vi "Udp Tester ffwd P Deadband.vi"() -> ()   [LabVIEW 2014]
uses:
  <vilib>/Simulation/Scripting/Companion Diagram/SimConfigNode/SimParams.ctl
  <vilib>/Simulation/Scripting/Companion Diagram/SimConfigNode/_simSolvers.ctl
  <vilib>/Simulation/Implementation/Shared/SIMSCR Execution Mode.ctl
  <vilib>/Platform/TimedLoop/XDataNode/timing_clust.ctl
  <vilib>/Platform/TimedLoop/XDataNode/nitl_modes.ctl
  <vilib>/Platform/TimedLoop/XDataNode/wakeup.ctl
  <vilib>/Simulation/Param Hierarchy/Typedefs/SIMPH Param Control Actions.ctl
  <vilib>/Simulation/Scripting/Editor Utilities/SIM subVI tag data.ctl
  <vilib>/Simulation/Scripting/Editor Utilities/SIM subVI execution type.ctl
  <vilib>/Simulation/Implementation/Shared/NILVSim_ParamChanged.vi
  <vilib>/Simulation/Implementation/Shared/NILVSim_FinishedLate.vi
  <vilib>/Simulation/Implementation/Shared/NILVSIM_BeginStep.vi
  <vilib>/Simulation/Utility/Implementation/SIM Time.vi
  <vilib>/Simulation/SignalArithmetic/Implementation/NILVSim Gain.llb/SIM Gain (scalar).vi
  <vilib>/Simulation/DiscreteLinear/Implementation/NILVSim Discrete Integrator Forward.llb/SIM Discrete Integrator Forward Distributor (scalar).vi
  <vilib>/Simulation/DiscreteLinear/Implementation/NILVSim Discrete Integrator Forward.llb/SIM Discrete Integrator Forward Collector (scalar).vi
  <vilib>/Simulation/DiscreteLinear/Implementation/NILVSim Discrete Transfer Function Buffered.llb/SIM Discrete Transfer Function Distributor (SISO).vi
  <vilib>/Simulation/DiscreteLinear/Implementation/NILVSim Discrete Transfer Function Direct.llb/SIM Discrete Transfer Function Direct (SISO).vi
  <vilib>/Simulation/Utility/Implementation/NILVSim Collector.llb/SIM Collector (vector).vi
  <vilib>/Simulation/SignalDisplay/Implementation/NILVSim Time Waveform.llb/SIM Time Waveform (vector).vi
  <vilib>/Simulation/Nonlinear/Implementation/NILVSim Saturation.llb/SIM Saturation (scalar).vi
  <vilib>/Simulation/ContinuousLinear/Implementation/NILVSim Transfer Function.llb/SIM Transfer Function Collector (SISO).vi
  <vilib>/Simulation/SignalDisplay/Implementation/NILVSim Time Waveform.llb/SIM Time Waveform (scalar).vi
  <vilib>/Simulation/Implementation/Shared/SIM Fire Discrete SubVI.vi
  <vilib>/Simulation/Implementation/Shared/NILVSim_Manager.vi
  <vilib>/Utility/error.llb/Clear Errors.vi
  <vilib>/Simulation/Implementation/Shared/NILVSim_FinalizeModel.vi
  <vilib>/Simulation/Utility/Implementation/NILVSim Collector.llb/NILVSim Collector core (vector).vi
  <vilib>/Simulation/Implementation/Shared/SIM Fire Discrete SubVI (Core).vi
  <vilib>/FPGAPlugInAG/myRIO-1900/niLvFpga_Open_myRIO-1900.vi
  <vilib>/rvi/interface/common/dynamic/niFpgaDynamicAddResources.vi
  <vilib>/Utility/error.llb/Error Cluster From Error Code.vi
  <vilib>/rvi/errors/niLvFpgaAdjustHostInterfaceError.vi
  <vilib>/FPGAPlugInAG/Dynamic/niLvFpga_Close_Dynamic.vi
  <vilib>/Simulation/Implementation/Shared/SIM Unbundle Sim Info.vi
  <vilib>/Simulation/Implementation/Shared/SIMSH Read Queue.vi
  <vilib>/Simulation/Implementation/Shared/NILVSim_Initialize.vi
  <vilib>/addons/Control Design/_Utility/Animation.llb/CD Time Delay Function.vi
  <vilib>/Simulation/Utility/Implementation/NILVSim Get Time and IsAcceptedStep.vi
  <vilib>/Utility/file.llb/Write To Spreadsheet File (DBL).vi
  <vilib>/Simulation/Implementation/Shared/NILVSim_GetModelError.vi
  <vilib>/Simulation/Implementation/Shared/SIM Bundle Sim Info.vi
  <vilib>/rvi/interface/nirviOpenFPGA/nirviOpenFPGA.xnode
  FPGA Bitfiles/Test_FPGATarget_CurrentControl_60eBuCSPTsI.lvbitx
  Current Control.vi
  <vilib>/rvi/interface/nirviReadWriteControl/nirviReadWriteControl.xnode
  <vilib>/rvi/interface/nirviCloseFPGA/nirviCloseFPGA.xnode
  <vilib>/Simulation/Scripting/Companion Diagram/SimConfigNode/SimDog.xnode
  <vilib>/Platform/TimedLoop/XDataNode/XDataNode.xnode
  <vilib>/Simulation/Implementation/XNodeFramework/SimXNode/SimX.xnode
  <vilib>/rvi/interface/Simulation/niFpgaSimulationCallBeginRW.vi
  NiFpgaLv.dll
  <vilib>/Simulation/DiscreteLinear/Implementation/NILVSim Discrete Transfer Function Buffered.llb/SIM Discrete Transfer Function Buffered (SISO).vi
  <vilib>/Simulation/DiscreteLinear/Implementation/NILVSim Discrete Integrator Forward.llb/SIM Discrete Integrator Forward (scalar).vi
  <vilib>/Utility/file.llb/Write To Spreadsheet File (I64).vi
  <vilib>/Platform/TimedLoop/XDataNode/XDNodeRunTimeDep.lvlib
  <vilib>/Simulation/Implementation/Shared/NI_SIM_Implementation.lvlib
panel:
  out "Error":errorcluster
  in  "Enclosing Tab":T1(tab)
  in  "Length (L)":dbl[unit]=4.0
  out "Height [h] (m)":dbl(slide)=0.9798385024498506 scale=0.0..2.0
  in  "STOP":bool
  in  "Setpoint":dbl(slide)=1.0 min=0.0 max=2.0 scale=0.0..0.75
  in  "Control Parameters":T2(tab)
  in  "Kpi 2":dbl(slide)=0.03 scale=0.01..5.0
  in  "Ki 2":dbl(slide)=0.03 scale=0.03897..0.0433
  in  "Kw":dbl(slide) scale=0.0..0.1
  in  "Kpd":dbl(slide)=0.03 scale=0.01..0.9
  out "Pump":bool=TRUE
  out "FT":dbl(knob)=84.28886007445381 scale=0.0..100.0
  out "Excitation":cluster{"Time":dbl[], "Signal":dbl[]}(graph)
  out "Response":cluster{"Time":dbl[], "Signal":dbl[]}(graph)
  out "Setpoint vs. IAB Height":waveform(dbl)[](graph)=[{"t0"=timestamp(1835.8000000000002 s since 1904-01-01), "dt"=1.0, "Y"=[0.9645428084016676]}, {"t0"=timestamp(1835.8000000000002 s since 1904-01-01), "dt"=1.0, "Y"=[1.0]}]
  out "Control Action":waveform(dbl)(graph)={"t0"=timestamp(1835.8000000000002 s since 1904-01-01), "dt"=1.0, "Y"=[0.011099999999999999]}
  out "Elapsed Time":dbl
  out "Current(mA)":dbl
  out "Static Response":cluster{dbl, "Input Signal":dbl}[](graph)
  out "Status?":bool
  # "LIC"
  # "101"
  # "LCV"
  # "101"
  # "LT"
  # "101"
  # "%"
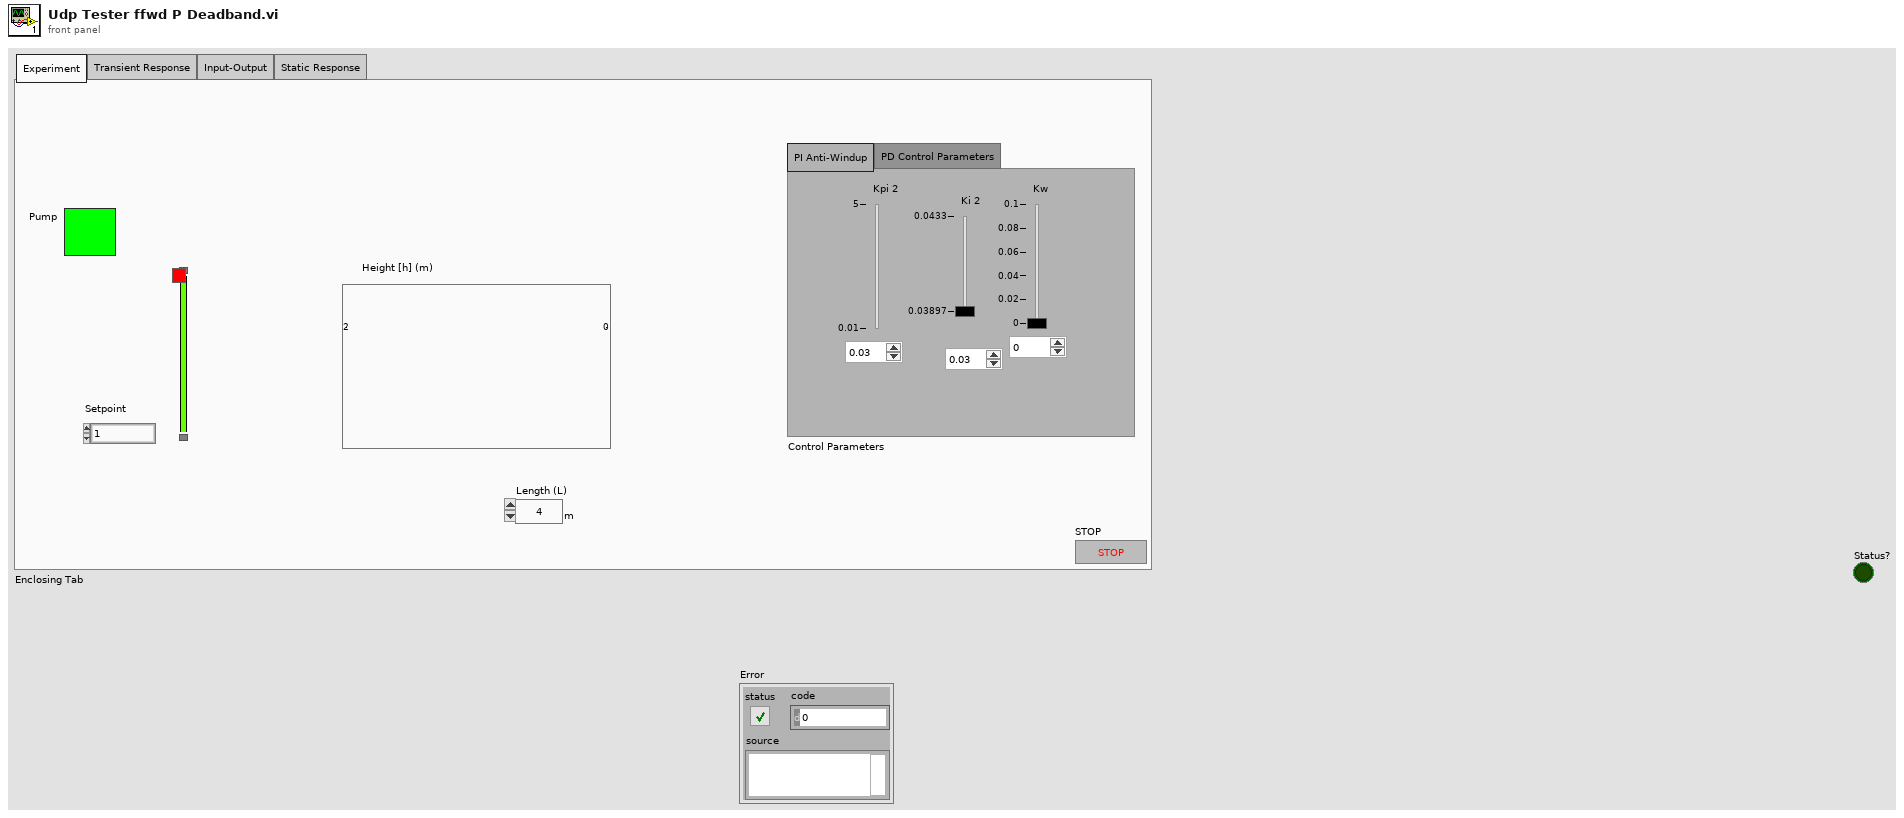
[diagram p1: front panel]
types:
  T1 = enum32{"Experiment", "Transient Response", "Input-Output", "Static Response"}
  T2 = enum32{"PI Anti-Windup", "PD Control Parameters"}
  T3 = enum16{"big-endian, network order", "native, host order", "little-endian"}
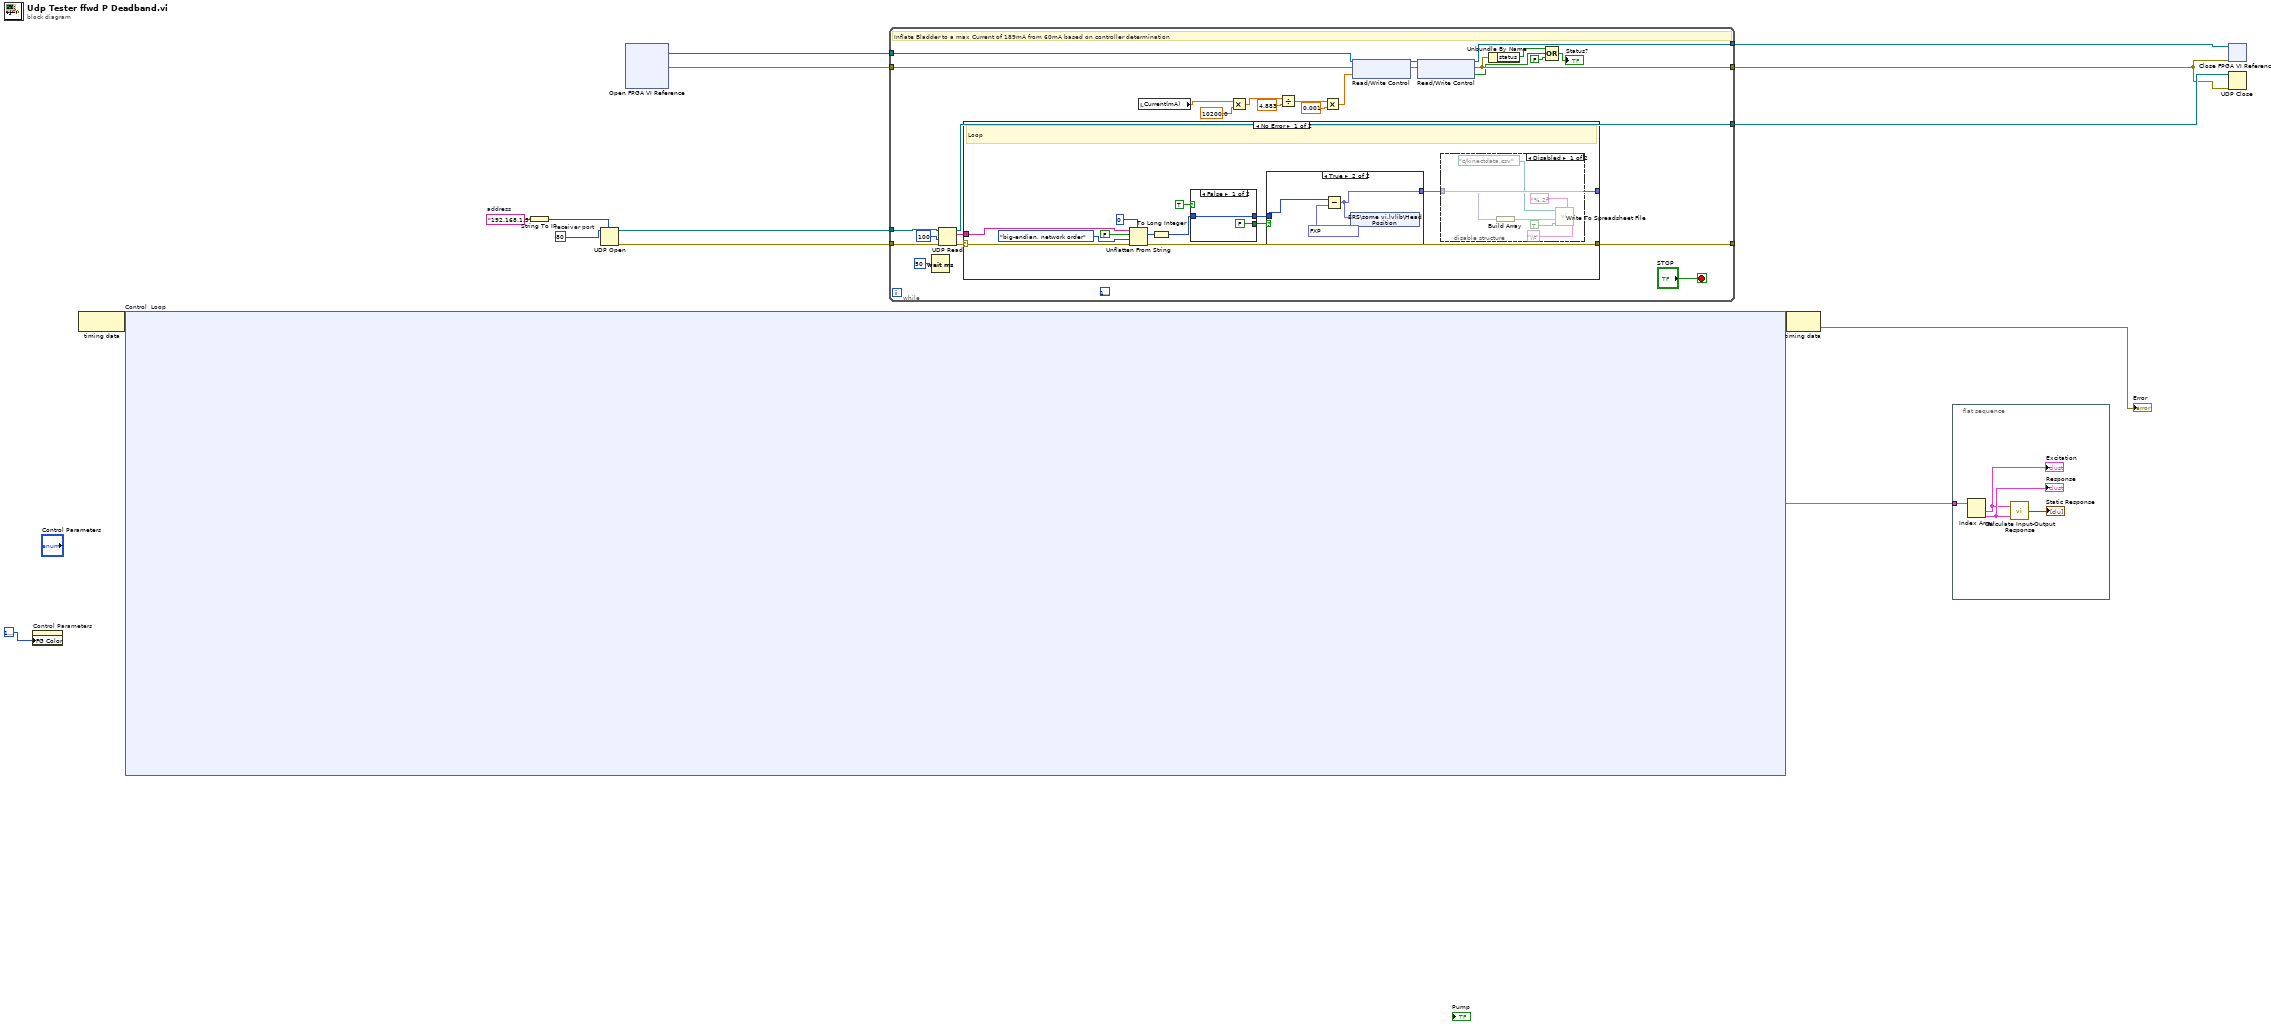
[diagram p0: block diagram]
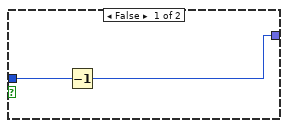
[diagram p3: hidden frame]
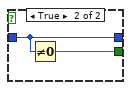
[diagram p4: hidden frame]
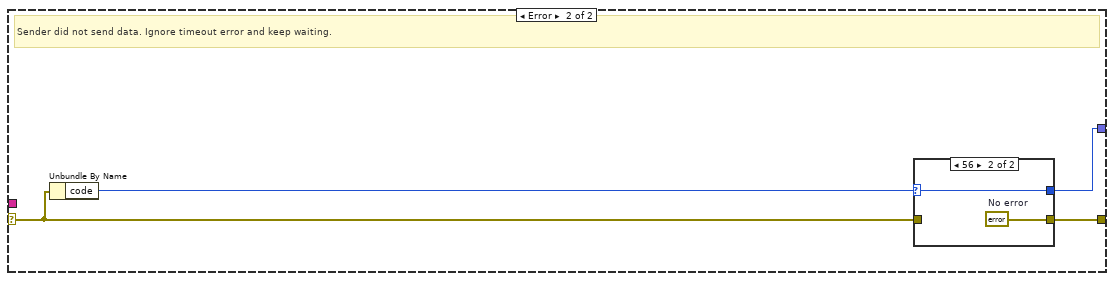
[diagram p5: hidden frame]
diagram:
  w14 = "192.168.1.5"  # address
  w13 = u16 80  # receiver port
  n1 = property on="Control Parameters" class="TabCtl (strict)"("FG Color"=u32 16777238) -> ()  [unwired: 2 in, 2 out]
  n2 = node-c288() -> (w5:variant)  [unwired: 1 in]
  n3 = node-c254 "Control  Loop"(w5) -> (w4:variant, w1:cluster{"Time":dbl[], "Signal":dbl[]}[])
  n4 = String To IP(1:w14) -> (0:w15:u32)
  n5 = UDP Open(7:w15, 11:w13) -> (port=w12:refnum<k16>, 0:w11:errorcluster)  [unwired: 3 in, 1 out]
  n6 = xnode "Open FPGA VI Reference"() -> ("FPGA VI Reference Out"=w7:refnum<k20>, "error out"=w6:errorcluster)  [unwired: 2 in]
  n7 = while {
    tunnel: w12 -> [w41]
    tunnel: w11 -> [w40]
    tunnel: w7 -> [w35]
    tunnel: [w36] -> w9
    tunnel: w6 -> [w38]
    tunnel: [w37] -> w8
    tunnel: [w20] -> _
    tunnel: [w19] -> w10
    stop <- "STOP" stop-if-true
    (unwired) u32 16777216
    # "Inflate Bladder to a max Current of 189mA from 60mA based on controller determination"
    n8 = Wait (ms)(milliseconds to wait=u32 50) -> ()  [unwired: 1 out]
    n9 = UDP Read(connection ID=w41, timeout ms (25000)=100, 8:w40) -> (data out=w22:string, error out=w21:errorcluster, 3:w19:refnum<k16>)  [unwired: 3 out]
    n10 = case shown="No Error" w21 {
      selector: w21 -> [w48 w71]
      tunnel: w22 -> [w49 _]
      tunnel: [w47 w70] -> w20
      tunnel: [w43 w69] -> _
      frame No Error {
        # "Loop"
        n11 = Unflatten From String(type=0, binary string=w49, data includes array or string size? (T)=FALSE, byte order (0:big-endian, network order)=T3."big-endian, network order" ("byte order"), error in (no error)=w48) -> (value=w50:i32, error out=w47:errorcluster)  [unwired: 1 out]
        n12 = To Long Integer(number=w50) -> (32bit integer=w45:i32)
        n13 = case shown="False" TRUE {
          tunnel: w45 -> [w65 w67]
          tunnel: [FALSE w68] -> w44
          tunnel: [w65 w67] -> w42
          frame False {
          }
          frame True {
            n14 = Not Equal To 0?(x=w67) -> (x != 0?=w68:bool)
          }
        }
        n15 = case shown="True" w44 {
          tunnel: w42 -> [w61 w63]
          tunnel: [w60 w62] -> w43
          frame False {
            n16 = Decrement(x=w61) -> (x-1=w60:i32)
          }
          frame True {
            n17 = Subtract(x=w63, y=fxp<+,18,8> 246.3818359375) -> (x-y=w62:fxp<+/-,43,33>)
            n18 = shared-variable "SRS\\some vi.lvlib\\Head Position"(w62) -> ()  [unwired: 1 in, 1 out]
          }
        }
        n19 = disable-structure shown="Disabled" {
          disable-tunnel: w43 -> [w54 _]
          frame Disabled {
            n20 = Build Array(w54) -> (w59:fxp<+/-,43,33>[])
            n21 = call-poly <vilib>:"Write To Spreadsheet File.vi"("delimiter (\\t)"="\\t" ("delimiter (\\t)"), "format (%d)"="%.2f", "append to file? (new file:F)"=TRUE, "1D data"=w59, "file path (dialog if empty)"=path "c:/kinectdata.csv") -> ()  [unwired: 3 in, 1 out]
          }
          frame Enabled {
          }
        }
      }
      frame Error {
        # "Sender did not send data. Ignore timeout error and keep waiting."
        n22 = Unbundle By Name(w71) -> ("code"=w72:i32)
        n23 = case shown="56" w72 {
          selector: w72 -> [w73 w75]
          tunnel: w71 -> [w74 _]
          tunnel: [w74 w76] -> w70
          tunnel: [w73 w75] -> w69
          frame Default {
          }
          frame 56 {
            w76 = errorcluster {"status"=FALSE, "code"=0, "source"=""}  # No error
          }
        }
      }
    }
    n24 = local read "Current(mA)"() -> (w16:dbl)
    n25 = Multiply(x=w16, y=10200.0) -> (x*y=w23:dbl)
    n26 = Divide(x=w23, y=4.883) -> (x/y=w26:dbl)
    n27 = Multiply(x=w26, y=0.001) -> (x*y=w32:dbl)
    n28 = xnode "Read/Write Control"("FPGA VI Reference In"=w35, "error in"=w38, "DAC Inlet Valve"=w32) -> ("FPGA VI Reference Out"=w34:refnum<k20>, "error out"=w33:errorcluster)
    n29 = xnode "Read/Write Control"("FPGA VI Reference In"=w34, "error in"=w33) -> ("FPGA VI Reference Out"=w36:refnum<k20>, "error out"=w37:errorcluster, "Inlet Overflow?"=w31:bool)
    n30 = Unbundle By Name(w37) -> ("status"=w29:bool)
    n31 = Compound Arithmetic op=OR(w29, w31, FALSE ("value")) -> (→"Status?":bool)
  }
  n32 = node-c288(w4) -> (→"Error":errorcluster)
  n33 = flat-sequence {
    tunnel: w1 -> [w78]
    frame #0 {
      n34 = Index Array(array=w78) -> (element #1=w77:cluster{"Time":dbl[], "Signal":dbl[]}, element #2=w80:cluster{"Time":dbl[], "Signal":dbl[]})  [unwired: 2 in]
      "Response" <- w80
      "Excitation" <- w77
      n35 = call "Calculate Input-Output Response.vi"("Response"=w80, "Input"=w77) -> ("Input-Output"=→"Static Response":cluster{dbl, "Input Signal":dbl}[])
    }
  }
  n36 = xnode "Close FPGA VI Reference"("FPGA VI Reference In"=w9, "error in"=w8) -> ()  [unwired: 1 out]
  n37 = UDP Close(connection ID=w10, 8:w8) -> ()  [unwired: 2 out]
